vi "Configure ACLR Measurement.vi"(0 "SA-FSW in":refnum<class "SA-FSW.lvclass">, 1 "TX Bandwidth [Hz]":dbl=100.0, 2 "TX Spacing [Hz]":dbl=14000.0, 3 "ALCR Type":enum16{"Relative [dBc]", "Absolute [dBm]"}(ring), 5 "TX Channels":i32=1, 9 "Adj Channels":i32=1, 11 "error in (no error)":errorcluster, 12 "Adj Bandwidth [Hz]":dbl, 13 "Adj Spacing [Hz]":dbl) -> (4 "SA-FSW out":refnum<class "SA-FSW.lvclass">, 15 "error out":errorcluster)   [LabVIEW 2020, in "SA-FSW.lvclass"]
uses:
  SA-FSW.lvclass
  C:/Sandbox/Git_Sandbox/WiSpry Test Framework source code (LV20)/WiSpry Test Framework/Instruments/Instrument.lvclass
  Instrument.lvclass/Instrument.ctl
  Instrument.lvclass
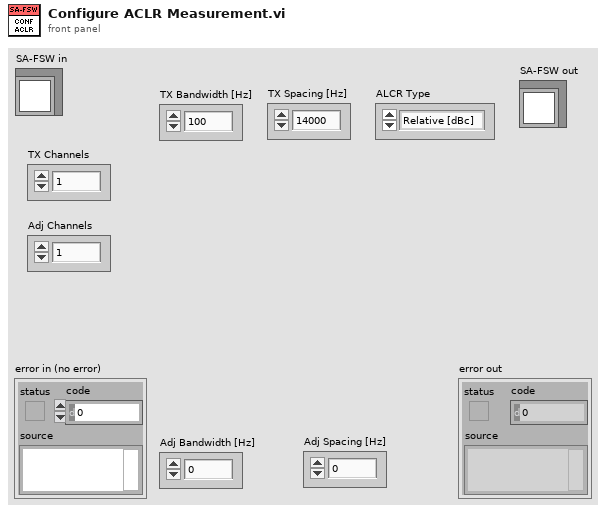
[diagram p1: front panel]
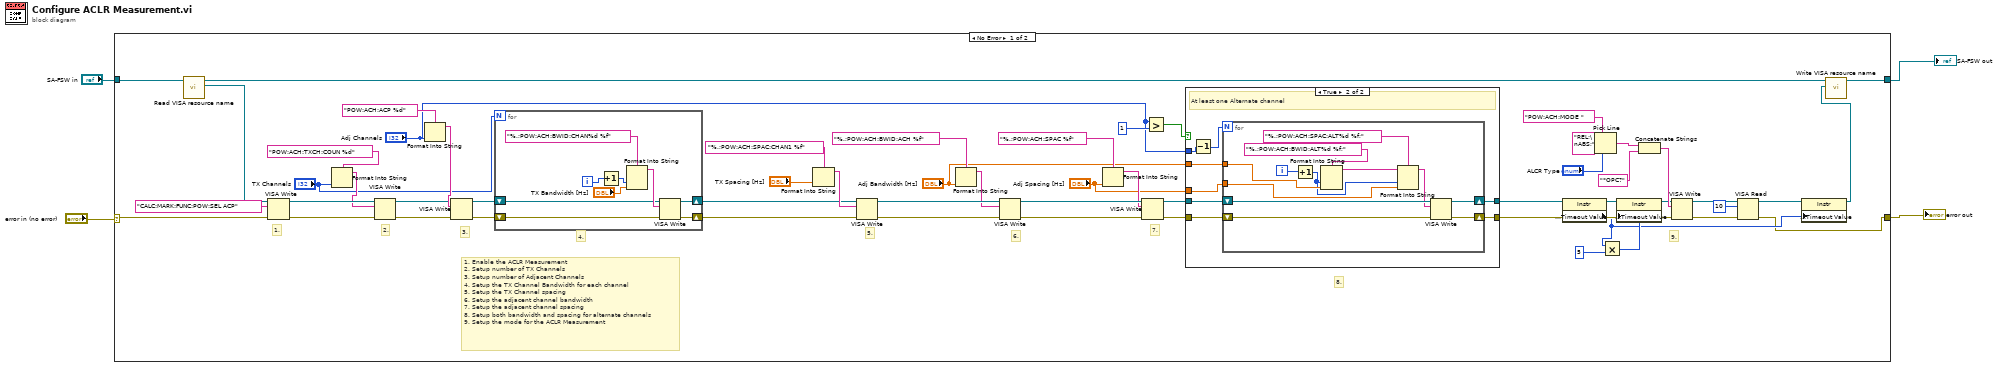
[diagram p0: block diagram]
diagram:
  n1 = case shown="No Error" "error in (no error)" {
    selector: "error in (no error)" -> [w59 w92]
    tunnel: "SA-FSW in" -> [w60 w93]
    tunnel: [w8 w92] -> w2
    tunnel: [w6 w93] -> w1
    frame No Error {
      # "9."
      # "8."
      # "7."
      # "6."
      # "5."
      # "4."
      # "1. Enable the ACLR Measurement\n2. Setup number of TX Channels\n3. Setup number of Adjacent Channels\n4. Setup the TX Channel Bandwidth for each channel\n5. Setup the TX Channel spacing\n6. Setup the adjacent channel bandwidth\n7. Setup the adjacent channel spacing\n8. Setup both bandwidth and spacing for alternate channels\n9. Setup the mode for the ACLR Measurement"
      # "3."
      # "2."
      # "1."
      n2 = call "Read VISA resource name.vi"("Instrument in"=w60) -> ("VISA resource name"=w58:refnum<visa-resource-name>, "Instrument out"=w7:refnum<class "SA-FSW.lvclass">)  [unwired: 9 in]
      n3 = VISA Write(VISA resource name=w58, write buffer="CALC:MARK:FUNC:POW:SEL ACP", error in (no error)=w59) -> (VISA resource name out=w55:refnum<visa-resource-name>, error out=w56:errorcluster)  [unwired: 1 out]
      n4 = Format Into String(format string="POW:ACH:TXCH:COUN %d" ("initial string"), "TX Channels") -> (resulting string=w54:string)  [unwired: 2 in, 1 out]
      n5 = VISA Write(VISA resource name=w55, write buffer=w54, error in (no error)=w56) -> (VISA resource name out=w51:refnum<visa-resource-name>, error out=w49:errorcluster)  [unwired: 1 out]
      n6 = Format Into String(format string="POW:ACH:ACP %d", "Adj Channels") -> (resulting string=w52:string)  [unwired: 2 in, 1 out]
      n7 = VISA Write(VISA resource name=w51, write buffer=w52, error in (no error)=w49) -> (VISA resource name out=w48:refnum<visa-resource-name>, error out=w47:errorcluster)  [unwired: 1 out]
      n8 = for {
        N: "TX Channels" -> [_]
        shift-right: [w87] -> w43
        shift-left: w48 -> [w89]
        shift-right: [w86] -> w42
        shift-left: w47 -> [w88]
        i -> [w83]
        n9 = Increment(x=w83) -> (x+1=w84:i32)
        n10 = Format Into String(format string="%.;POW:ACH:BWID:CHAN%d %f", w84, "TX Bandwidth [Hz]") -> (resulting string=w90:string)  [unwired: 2 in, 1 out]
        n11 = VISA Write(VISA resource name=w89, write buffer=w90, error in (no error)=w88) -> (VISA resource name out=w87:refnum<visa-resource-name>, error out=w86:errorcluster)  [unwired: 1 out]
      }
      n12 = Format Into String(format string="%.;POW:ACH:SPAC:CHAN1 %f", "TX Spacing [Hz]") -> (resulting string=w44:string)  [unwired: 2 in, 1 out]
      n13 = VISA Write(VISA resource name=w43, write buffer=w44, error in (no error)=w42) -> (VISA resource name out=w39:refnum<visa-resource-name>, error out=w37:errorcluster)  [unwired: 1 out]
      n14 = Format Into String(format string="%.;POW:ACH:BWID:ACH %f", "Adj Bandwidth [Hz]") -> (resulting string=w38:string)  [unwired: 2 in, 1 out]
      n15 = VISA Write(VISA resource name=w39, write buffer=w38, error in (no error)=w37) -> (VISA resource name out=w34:refnum<visa-resource-name>, error out=w35:errorcluster)  [unwired: 1 out]
      n16 = Format Into String(format string="%.;POW:ACH:SPAC %f", "Adj Spacing [Hz]") -> (resulting string=w33:string)  [unwired: 2 in, 1 out]
      n17 = VISA Write(VISA resource name=w34, write buffer=w33, error in (no error)=w35) -> (VISA resource name out=w28:refnum<visa-resource-name>, error out=w32:errorcluster)  [unwired: 1 out]
      n18 = Greater?(x="Adj Channels", y=1) -> (0:w31:bool)
      n19 = case shown="True" w31 {
        tunnel: w32 -> [w62 w70]
        tunnel: "Adj Channels" -> [_ w68]
        tunnel: w28 -> [w61 w69]
        tunnel: "Adj Bandwidth [Hz]" -> [_ w66]
        tunnel: "Adj Spacing [Hz]" -> [_ w65]
        tunnel: [w62 w64] -> w22
        tunnel: [w61 w63] -> w15
        frame False {
          # "No Alternate channel"
        }
        frame True {
          # "At least one Alternate channel"
          n20 = Decrement(x=w68) -> (x-1=w67:i32)
          n21 = for {
            N: w67 -> [_]
            shift-right: [w71] -> w64
            shift-left: w70 -> [w79]
            shift-right: [w72] -> w63
            shift-left: w69 -> [w78]
            tunnel: w66 -> [w80]
            tunnel: w65 -> [w74]
            i -> [w82]
            n22 = Increment(x=w82) -> (x+1=w75:i32)
            n23 = Format Into String(format string="%.;POW:ACH:BWID:ALT%d %f;", w75, w80) -> (resulting string=w77:string)  [unwired: 2 in, 1 out]
            n24 = Format Into String(format string="%.;POW:ACH:SPAC:ALT%d %f;", initial string=w77, w75, w74) -> (resulting string=w73:string)  [unwired: 1 in, 1 out]
            n25 = VISA Write(VISA resource name=w78, write buffer=w73, error in (no error)=w79) -> (VISA resource name out=w72:refnum<visa-resource-name>, error out=w71:errorcluster)  [unwired: 1 out]
          }
        }
      }
      n26 = property class="Instr"(reference=w15) -> (reference out=w13:refnum<visa-resource-name>, "General Settings:Timeout Value"=w9:u32)  [unwired: 1 in, 1 out]
      n27 = Pick Line(string ("")="POW:ACH:MODE ", multi-line string="REL;\nABS;", line index="ALCR Type") -> (output string=w21:string)
      n28 = Multiply(x=w9, y=u32 5) -> (x*y=w12:u32)
      n29 = property class="Instr"(reference=w13, "General Settings:Timeout Value"=w12) -> (reference out=w14:refnum<visa-resource-name>)  [unwired: 1 in, 1 out]
      n30 = Concatenate Strings(w21, "*OPC?" ("string")) -> (w20:string)
      n31 = VISA Write(VISA resource name=w14, write buffer=w20, error in (no error)=w22) -> (VISA resource name out=w17:refnum<visa-resource-name>, error out=w18:errorcluster)  [unwired: 1 out]
      n32 = VISA Read(VISA resource name=w17, byte count=u32 10, error in (no error)=w18) -> (VISA resource name out=w10:refnum<visa-resource-name>, error out=w8:errorcluster)  [unwired: 2 out]
      n33 = property class="Instr"(reference=w10, "General Settings:Timeout Value"=w9) -> (reference out=w5:refnum<visa-resource-name>)  [unwired: 1 in, 1 out]
      n34 = call "Write VISA resource name.vi"("VISA resource name"=w5, "Instrument in"=w7) -> ("Instrument out"=w6:refnum<class "SA-FSW.lvclass">)  [unwired: 9 in]
    }
    frame Error {
    }
  }
  "error out" <- w2
  "SA-FSW out" <- w1
